vi "Print.vi"(8 "error in (no error)":errorcluster, 9 "Line":string, 11 "reference in":refnum<class "Console.lvclass">) -> (0 "error out":errorcluster, 3 "reference out":refnum<class "Console.lvclass">)   [LabVIEW 2018, in "Console.lvclass"]
doc: "Print a line to the console"
uses:
  Console.lvclass
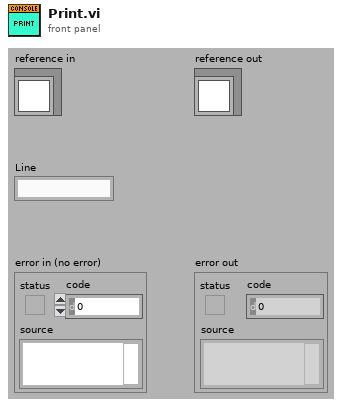
[diagram p1: front panel]
types:
  T1 = typedef "Console.lvclass/ObjectAttributes.ctl" = cluster{"data":string, "count":dbl}
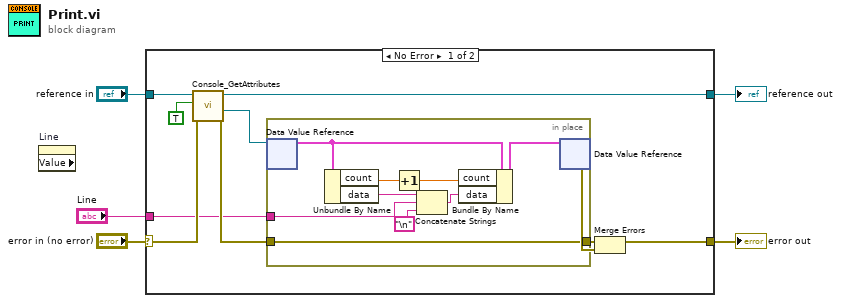
[diagram p0: block diagram]
diagram:
  n1 = property on="Line" class="Str" props=["Value"]() -> ()  [unwired: 2 in, 3 out]
  n2 = case shown="No Error" "error in (no error)" {
    selector: "error in (no error)" -> [w12 w26]
    tunnel: [w7 w26] -> w4
    tunnel: [w6 w25] -> w2
    tunnel: "reference in" -> [w14 w25]
    tunnel: "Line" -> [w8 _]
    frame No Error {
      n3 = call "Console_GetAttributes.vi"("error in (no error)"=w12, "OnlyGetDvrReference(False)"=TRUE, "reference in"=w14) -> ("error out"=w11:errorcluster, "DataRef"=w13:refnum<data-value>, "reference out"=w6:refnum<class "Console.lvclass">)  [unwired: 5 in, 1 out]
      n4 = in-place {
        in-place-border: w11 -> [w23]
        in-place-border: [w23] -> w10
        in-place-border: w8 -> [w19]
        n5 = in-place-dvr #1(w13) -> (w22:T1)  [unwired: 1 out]
        n6 = Unbundle By Name(w22) -> ("count"=w17:dbl, "data"=w21:string)
        n7 = Increment(x=w17) -> (x+1=w16:dbl)
        n8 = Concatenate Strings(w21, w19, "\n") -> (w20:string)
        n9 = Bundle By Name(cluster=w22, "count"=w16, "data"=w20) -> (w24:T1)
        n10 = in-place-dvr #1(w24) -> (w15:errorcluster)  [unwired: 1 out]
      }
      n11 = Merge Errors(w10, w15) -> (w7:errorcluster)
    }
    frame Error {
    }
  }
  "error out" <- w4
  "reference out" <- w2
